vi "Ping.vi"(6 "timeout (ms)":i32=500, 8 "error in (no error)":errorcluster, 11 "ip or hostname":string) -> (0 "error out":errorcluster, 1 "status":i32(ring) items=["Success"=0, "DestinationNetworkUnreachable"=11002, "DestinationHostUnreachable"=11003, "DestinationProhibited, DestinationProtocolUnreachable"=11004, "DestinationPortUnreachable"=11005, "NoResources"=11006, "BadOption"=11007, "HardwareError"=11008, "PacketTooBig"=11009, "TimedOut"=11010, "BadRoute"=11012, "TtlExpired"=11013, "TtlReassemblyTimeExceeded"=11014, "ParameterProblem"=11015, "SourceQuench"=11016, "BadDestination"=11018, "DestinationUnreachable"=11040, "TimeExceeded"=11041, "BadHeader"=11042, "UnrecognizedNextHeader"=11043, "IcmpError"=11044, "DestinationScopeMismatch"=11045, "Unknown"=-1], 2 "roundtrip time":i64, 3 "OK":bool)   [LabVIEW 2017, in "Windows Networking.lvlib"]
uses:
  Windows Networking.lvlib
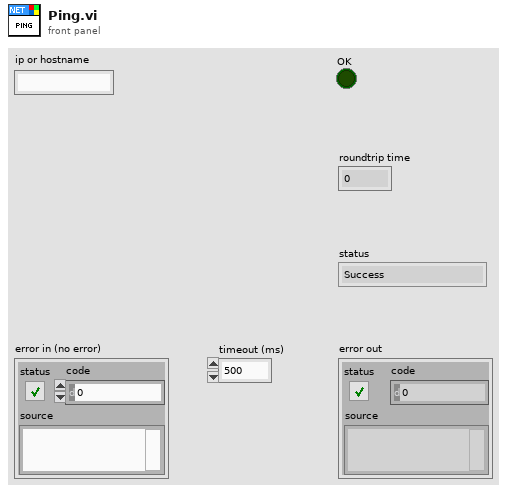
[diagram p1: front panel]
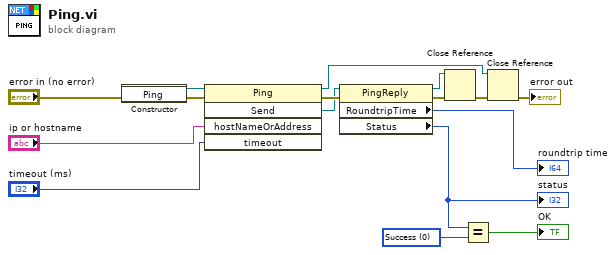
[diagram p0: block diagram]
diagram:
  w5 = 0 items=["Success"=0, "DestinationNetworkUnreachable"=11002, "DestinationHostUnreachable"=11003, "DestinationProhibited, DestinationProtocolUnreachable"=11004, "DestinationPortUnreachable"=11005, "NoResources"=11006, "BadOption"=11007, "HardwareError"=11008, "PacketTooBig"=11009, "TimedOut"=11010, "BadRoute"=11012, "TtlExpired"=11013, "TtlReassemblyTimeExceeded"=11014, "ParameterProblem"=11015, "SourceQuench"=11016, "BadDestination"=11018, "DestinationUnreachable"=11040, "TimeExceeded"=11041, "BadHeader"=11042, "UnrecognizedNextHeader"=11043, "IcmpError"=11044, "DestinationScopeMismatch"=11045, "Unknown"=-1] ("status 2")
  n1 = constructor class="Ping"(error in="error in (no error)") -> (reference out=w15:refnum<k24>, error out=w14:errorcluster)  [unwired: 2 in, 1 out]
  n2 = invoke class="Ping" method="Send"(reference=w15, error in=w14, "hostNameOrAddress"="ip or hostname", "timeout"="timeout (ms)") -> (reference out=w8:refnum<k24>, error out=w16:errorcluster, "Send"=w9:refnum<k24>)  [unwired: 1 in, 2 out]
  n3 = property class="PingReply"(reference=w9, error in=w16) -> (reference out=w2:refnum<k24>, error out=w3:errorcluster, "RoundtripTime"=→"roundtrip time":i64, "Status"=w6:i32)
  "status" <- w6
  n4 = Close Reference(reference=w2, error in (no error)=w3) -> (error out=w1:errorcluster)
  n5 = Equal?(x=w6, y=w5) -> (x = y?=→"OK":bool)
  n6 = Close Reference(reference=w8, error in (no error)=w1) -> (error out=→"error out":errorcluster)
